vi "LIght sensor code.vi"   [LabVIEW 2016, in "Ourbot.lvrbt"]
uses:
  Ourbot.lvrbt
  <vilib>/NXT/Block Support/NXT_ButtonSelector.ctl
  <vilib>/NXT/Block Support/NXT_InputPort.ctl
  <vilib>/NXT/Block Support/NXT_OutputPort.ctl
  <vilib>/NXT/Dual Mode Library/Sensors/readNXTButton.vi
  <vilib>/NXT/NXTIO Xnodes/NXTIONodeSubVIs/NXTMoveMotors.vi
  <vilib>/NXT/Dual Mode Library/Waits/Wait_Num(msec).vi
  <vilib>/NXT/Dual Mode Library/Sensors/EV3_Color_Ambient.vi
  <vilib>/NXT/Dual Mode Library/Waits/Wait_Num.vi
  <vilib>/NXT/Dual Mode Library/Waits/Wait_EV3_Color_Ambient_Greater.vi
  <vilib>/NXT/Subs/LVHSConnector.ctl
  <vilib>/NXT/NXTIO Xnodes/AddressXNode/NXTIOAddress.xnode
  <vilib>/NXT/NXTIO Xnodes/NXTIOXNode/NXTIO.xnode
  <vilib>/NXT/LegoClasses/BrickReference/BrickReference.lvclass
types:
  T1 = typedef "NXT_OutputPort.ctl" = u8
  T2 = typedef "NXT_InputPort.ctl" = u32
  T3 = typedef "NXT_ButtonSelector.ctl" = u16
  T4 = typedef "LVHSConnector.ctl" = refnum<class "BrickReference.lvclass">
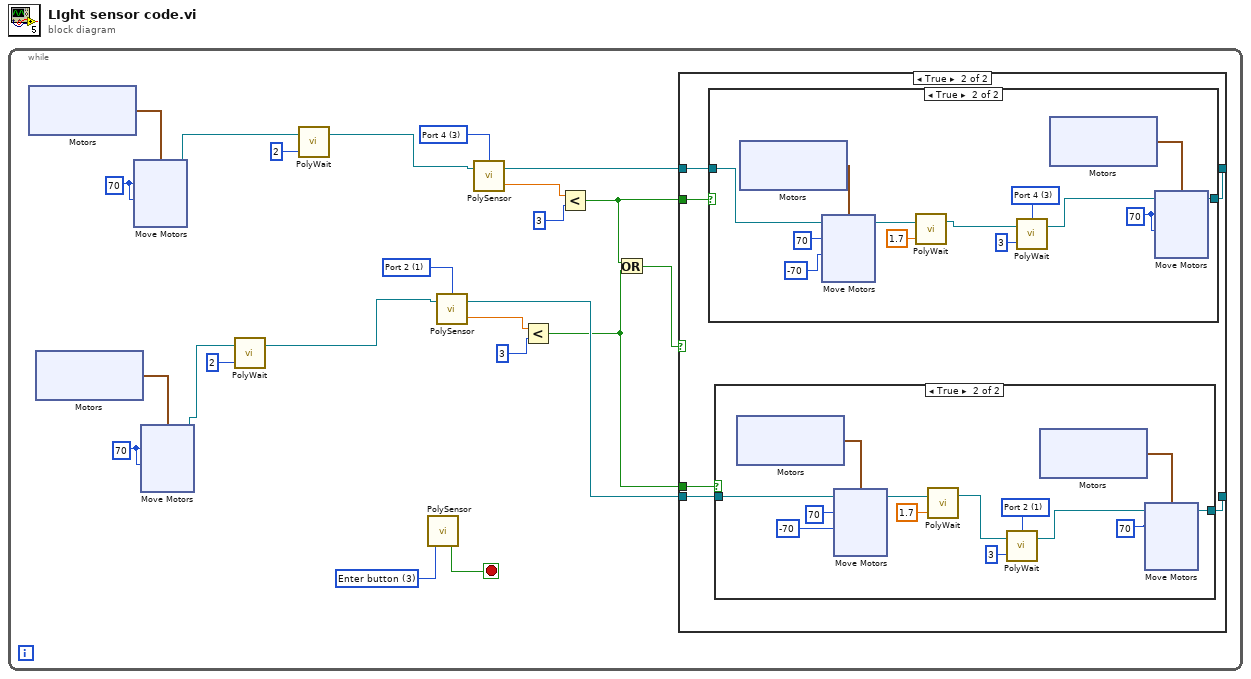
[diagram p0: block diagram]
diagram:
  n1 = while {
    stop <- w20 stop-if-true
    w8 = T2 3 items=["Port 1", "Port 2", "Port 3", "Port 4"] ("Port (Port 1)")
    w11 = T2 1 items=["Port 1", "Port 2", "Port 3", "Port 4"] ("Port (Port 1)")
    w16 = 70
    w19 = T3 3 items=["Enter button"=3, "Left button"=2, "Right button"=1, "Up Button"=4, "Down Button"=5] ("Button (Enter button)")
    w18 = 70
    n2 = xnode "Motors"() -> ("Motor"=w22:cluster{"Port":T1, "Port":T1})
    n3 = xnode "Motors"() -> ("Motor"=w17:cluster{"Port":T1, "Port":T1})
    n4 = xnode "Move Motors"("Power/Speed 2"=w18, "Power/Speed 1"=w18, "Motors"=w22) -> ("NXT/EV3"=w21:T4)  [unwired: 1 in]
    n5 = xnode "Move Motors"("Power/Speed 2"=w16, "Power/Speed 1"=w16, "Motors"=w17) -> ("NXT/EV3"=w14:T4)  [unwired: 1 in]
    n6 = call-poly <vilib>:"PolyWait.vi"("Time (100 msec)"=2, "NXT/EV3"=w14) -> ("NXT/EV3"=w12:T4)  [unwired: 2 in]
    n7 = call-poly <vilib>:"PolyWait.vi"("Time (100 msec)"=2, "NXT/EV3"=w21) -> ("NXT/EV3"=w6:T4)  [unwired: 2 in]
    n8 = call-poly <vilib>:"PolySensor.vi"("Button (Enter button)"=w19) -> ("Yes/No"=w20:bool)  [unwired: 2 in, 1 out]
    n9 = call-poly <vilib>:"PolySensor.vi"("NXT/EV3"=w12, "Port (Port 1)"=w11) -> ("Scaled Value"=w13:sgl, "NXT/EV3"=w4:T4)  [unwired: 1 in]
    n10 = call-poly <vilib>:"PolySensor.vi"("NXT/EV3"=w6, "Port (Port 1)"=w8) -> ("Scaled Value"=w9:sgl, "NXT/EV3"=w5:T4)  [unwired: 1 in]
    n11 = Less?(x=w13, y=3) -> (x < y?=w1:bool)
    n12 = Less?(x=w9, y=3) -> (x < y?=w2:bool)
    n13 = Or(x=w2, y=w1) -> (x .or. y?=w3:bool)
    n14 = case shown="True" w3 {
      tunnel: w5 -> [w25 w31]
      tunnel: w4 -> [w24 w30]
      tunnel: w2 -> [_ w29]
      tunnel: w1 -> [_ w28]
      tunnel: [w25 w27] -> _
      tunnel: [w24 w26] -> _
      frame False {
      }
      frame True {
        n15 = case shown="True" w29 {
          tunnel: w31 -> [w64 w66]
          tunnel: [w64 w65] -> w27
          frame False {
          }
          frame True {
            w68 = 70
            w73 = T2 3 items=["Port 1", "Port 2", "Port 3", "Port 4"] ("Port (Port 1)")
            n16 = xnode "Motors"() -> ("Motor"=w74:cluster{"Port":T1, "Port":T1})
            n17 = xnode "Move Motors"("Power/Speed 2"=-70, "Power/Speed 1"=70, "Motors"=w74, "NXT/EV3"=w66) -> ("NXT/EV3"=w77:T4)
            n18 = call-poly <vilib>:"PolyWait.vi"("Time (1 sec)"=1.7, "NXT/EV3"=w77) -> ("NXT/EV3"=w71:T4)  [unwired: 2 in]
            n19 = call-poly <vilib>:"PolyWait.vi"("Scaled Value (30)"=3, "NXT/EV3"=w71, "Port (Port 1)"=w73) -> ("NXT/EV3"=w69:T4)  [unwired: 1 in]
            n20 = xnode "Motors"() -> ("Motor"=w70:cluster{"Port":T1, "Port":T1})
            n21 = xnode "Move Motors"("Power/Speed 2"=w68, "Power/Speed 1"=w68, "Motors"=w70, "NXT/EV3"=w69) -> ("NXT/EV3"=w65:T4)
          }
        }
        n22 = case shown="True" w28 {
          tunnel: w30 -> [w32 w34]
          tunnel: [w32 w33] -> w26
          frame False {
          }
          frame True {
            w36 = 70
            w41 = T2 1 items=["Port 1", "Port 2", "Port 3", "Port 4"] ("Port (Port 1)")
            n23 = xnode "Motors"() -> ("Motor"=w42:cluster{"Port":T1, "Port":T1})
            n24 = xnode "Move Motors"("Power/Speed 1"=70, "Motors"=w42, "NXT/EV3"=w34, "Power/Speed 2"=-70) -> ("NXT/EV3"=w45:T4)
            n25 = call-poly <vilib>:"PolyWait.vi"("Time (1 sec)"=1.7, "NXT/EV3"=w45) -> ("NXT/EV3"=w37:T4)  [unwired: 2 in]
            n26 = call-poly <vilib>:"PolyWait.vi"("Scaled Value (30)"=3, "NXT/EV3"=w37, "Port (Port 1)"=w41) -> ("NXT/EV3"=w38:T4)  [unwired: 1 in]
            n27 = xnode "Motors"() -> ("Motor"=w39:cluster{"Port":T1, "Port":T1})
            n28 = xnode "Move Motors"("Power/Speed 2"=w36, "Power/Speed 1"=w36, "Motors"=w39, "NXT/EV3"=w38) -> ("NXT/EV3"=w33:T4)
          }
        }
      }
    }
  }
